vi "SetJogParameters.vi"(8 "error in (no error)":errorcluster, 10 "Jog Parameters":T1, 11 "KIM101 in":refnum<class "KIM101.lvclass">) -> (0 "error out":errorcluster, 3 "KIM101 out":refnum<class "KIM101.lvclass">)   [LabVIEW 2023, in "KIM101.lvlib" / "KIM101.lvclass"]
uses:
  KIM101.lvclass
  KIM101.lvlib
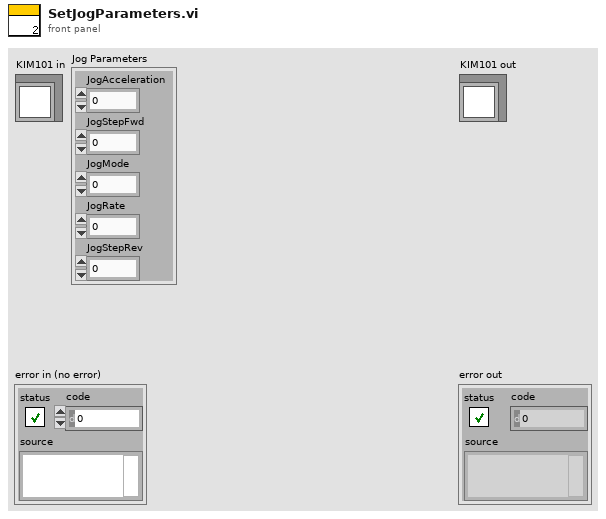
[diagram p1: front panel]
types:
  T1 = cluster{"JogAcceleration":i32, "JogStepFwd":i32, "JogMode":i32, "JogRate":i32, "JogStepRev":i32}
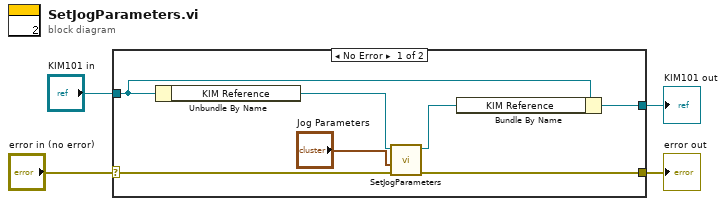
[diagram p0: block diagram]
diagram:
  n1 = case shown="No Error" "error in (no error)" {
    selector: "error in (no error)" -> [w7 w13]
    tunnel: [w6 w13] -> w3
    tunnel: [w9 w12] -> w1
    tunnel: "KIM101 in" -> [w8 w12]
    frame No Error {
      n2 = Unbundle By Name(w8) -> ("KIM Reference"=w11:refnum<k24>)
      n3 = call "SetJogParameters.vi"("error in (no error)"=w7, "Jog Parameters"="Jog Parameters", "KIM Reference"=w11) -> ("error out"=w6:errorcluster, "KIM Reference"=w10:refnum<k24>)  [unwired: 7 in]
      n4 = Bundle By Name(cluster=w8, "KIM Reference"=w10) -> (w9:refnum<class "KIM101.lvclass">)
    }
    frame Error {
    }
  }
  "error out" <- w3
  "KIM101 out" <- w1
